vi "Obtain Trigger Queue.vi"(0 "trigger queue name":string, 11 "error in":errorcluster) -> (4 "trigger queue out":refnum<queue>, 15 "error out":errorcluster)   [LabVIEW 2023, in "TLB` InstStu GPlugin Template.lvlib" / "{TMPL} Trigger API.lvlib"]
doc: "Create trigger queue resource for communication.\n\n<B>Input Parameters</B>\n\n<B>trigger queue name</B> specific action queue name.\n\n<B>error in</B> describes error conditions that occur before this node runs. This input provides standard error in functionality.\n\n<B>Output Parameters</B>\n\n<B>trigger queue out</B> is a reference to the existing queue or the new queue created by this function.\n\n<B>error out</B> contains error information. This output provides standard error out functionality."
uses:
  {TMPL} Trigger API.lvlib
  System Trigger Element.ctl
  System Trigger.ctl
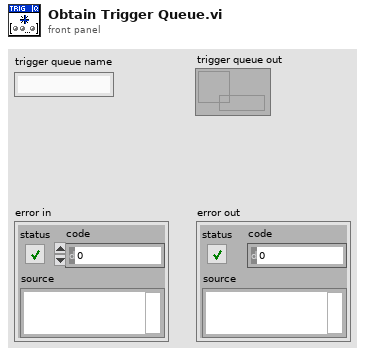
[diagram p1: front panel]
types:
  T1 = typedef "TLB` InstStu GPlugin Template.lvlib/{TMPL} Trigger API.lvlib/System Trigger Element.ctl" = cluster{"System Trigger":T2, "Trigger Data":variant}
  T2 = typedef "TLB` InstStu GPlugin Template.lvlib/{TMPL} Trigger API.lvlib/System Trigger.ctl" = enum16{"<None>", "Connect", "Start Acquisition", "Stop Acquisition", "Disconnect", "Load Configuration", "Save Configuration", "<Return to Safe State Actions>", "<Cache User Parameters>", "<Close Application>", "<Error>"}
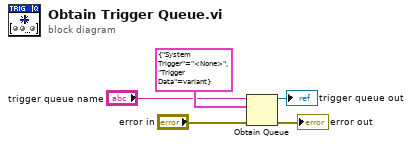
[diagram p0: block diagram]
diagram:
  n1 = Obtain Queue(name (unnamed)="trigger queue name", element data type=T1 {"System Trigger"=enum."<None>", "Trigger Data"=variant} ("element"), error in (no error)="error in") -> (queue out=→"trigger queue out":refnum<queue>, error out=→"error out":errorcluster)  [unwired: 2 in, 1 out]
